vi "Load 1.vi"(0 "LV MDI in":refnum<class "LV MDI.lvclass">, 5 "Vi Path":path=path "C:/Users/namratha.balakrishna/Documents/LabVIEW Data/MDI/source code/Labview MDI/Example/Waveform.vi", 11 "error in (no error)":errorcluster) -> (4 "LV MDI out":refnum<class "LV MDI.lvclass">, 6 "Name[]":string[](array[string]), 15 "error out":errorcluster)   [LabVIEW 2016]
doc: "Stores the VI reference,FP title,Hwnd in memory."
uses:
  LV Doc.lvclass
  LV MDI.lvclass
  D:/MDI Project/source code/API/MDI_Class/Document.lvclass
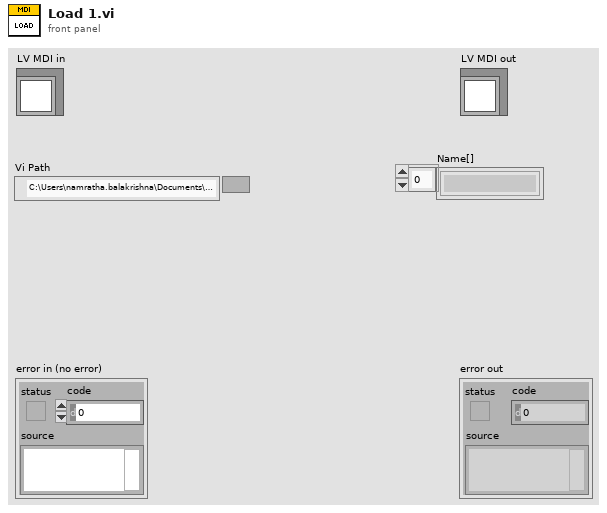
[diagram p1: front panel]
types:
  T1 = typedef "LV MDI.lvclass/Child Window Data.ctl" = cluster{"Child hWnd":u32, "UID":string, "vi reference":refnum<vi>, "Name":string}
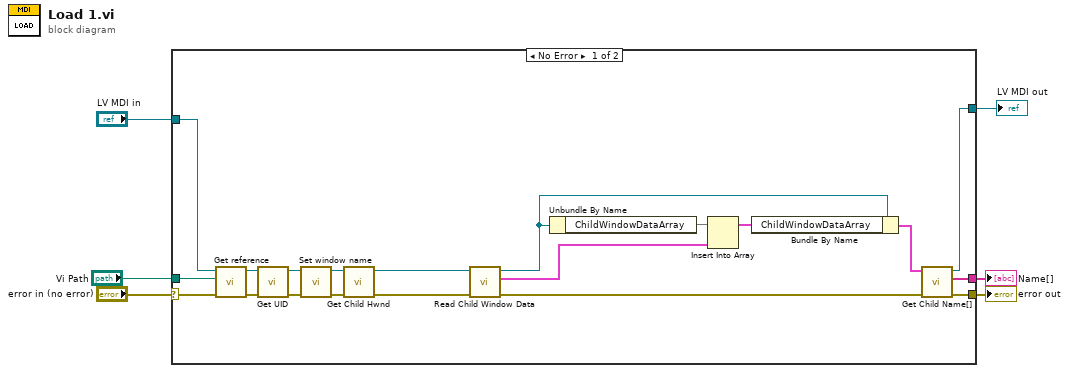
[diagram p0: block diagram]
diagram:
  n1 = case shown="No Error" "error in (no error)" {
    selector: "error in (no error)" -> [w25 w28]
    tunnel: [w10 w28] -> w5
    tunnel: [w8 w27] -> w3
    tunnel: "LV MDI in" -> [w23 w27]
    tunnel: "Vi Path" -> [w24 _]
    tunnel: [w7 _] -> w1
    frame No Error {
      n2 = call "Get reference.vi"("Error in"=w25, "Vi Path"=w24, "LV Doc.lvclass"=w23) -> ("Error Out"=w26:errorcluster, "LV Doc.lvclass"=w22:refnum<class "LV Doc.lvclass">)  [unwired: 7 in]
      n3 = call "Get UID.vi"("error in (no error)"=w26, "LV Doc.lvclass"=w22) -> ("error out"=w20:errorcluster, "LV Doc.lvclass"=w21:refnum<class "LV Doc.lvclass">)  [unwired: 8 in]
      n4 = call "Set window name.vi"("error in (no error)"=w20, "LV Doc.lvclass"=w21) -> ("error out"=w15:errorcluster, "LV Doc.lvclass"=w16:refnum<class "LV Doc.lvclass">)  [unwired: 8 in]
      n5 = call "Get Child Hwnd.vi"("Error in"=w15, "LV Doc.lvclass"=w16) -> ("Error Out"=w13:errorcluster, "LV Doc.lvclass"=w14:refnum<class "LV Doc.lvclass">)  [unwired: 8 in]
      n6 = call-dynamic "Read Child Window Data.vi"("error in (no error)"=w13, "LV MDI.lvclass"=w14) -> ("error out"=w19:errorcluster, "Child Window Data"=w12:T1, "LV MDI.lvclass"=w17:refnum<class "LV MDI.lvclass">)  [unwired: 7 in]
      n7 = Unbundle By Name(w17) -> ("ChildWindowDataArray"=w18)
      n8 = Insert Into Array(array=w18, new element=w12) -> (w11:T1[])  [unwired: 1 in]
      n9 = Bundle By Name(cluster=w17, "ChildWindowDataArray"=w11) -> (w9:cluster{})
      n10 = call "Get Child Name[].vi"("error in (no error)"=w19, "LV Doc.lvclass"=w9) -> ("error out"=w10:errorcluster, "Array"=w7:string[], "LV Doc.lvclass"=w8:refnum<class "LV Doc.lvclass">)  [unwired: 7 in]
    }
    frame Error {
    }
  }
  "error out" <- w5
  "LV MDI out" <- w3
  "Name[]" <- w1
